vi "fgv_Gslam_history.vi"(7 "cmd":T1, 9 "z":dbl[][](array[numeric]), 10 "x_dr":cluster{"x":dbl, "y":dbl, "yaw":dbl}, 11 "x_true":cluster{"x":dbl, "y":dbl, "yaw":dbl}) -> (1 "hz":dbl[][][](array[numeric]), 2 "hxDR":cluster{"x":dbl, "y":dbl, "yaw":dbl}[](array[cluster]), 3 "hxTrue":cluster{"x":dbl, "y":dbl, "yaw":dbl}[](array[cluster]))   [LabVIEW 2019]
uses:
  Ctrl/mbuffer.ctl
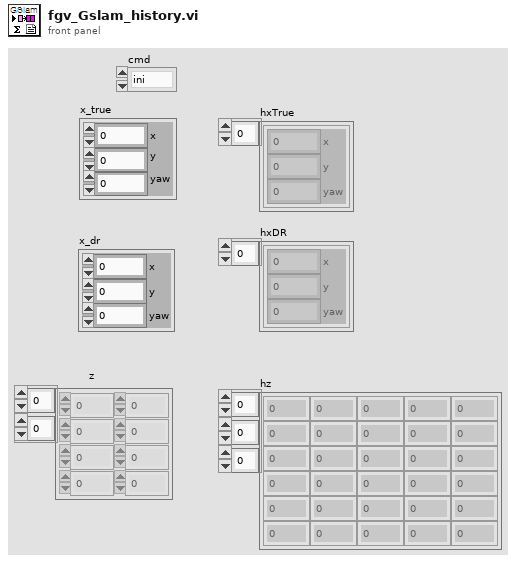
[diagram p1: front panel]
types:
  T1 = typedef "mbuffer.ctl" = enum16{"ini", "add", "read"}
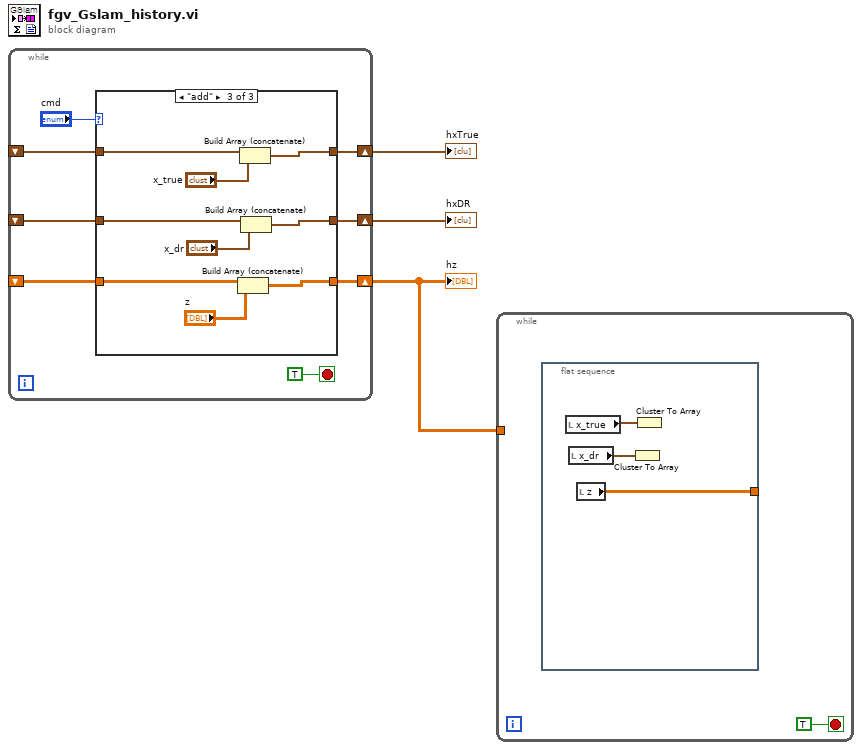
[diagram p0: block diagram]
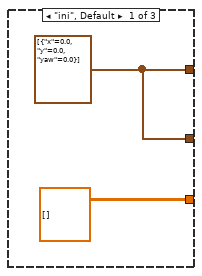
[diagram p2: hidden frame]
diagram:
  n1 = while {
    shift-right: [w10] -> w2
    shift-left: _ -> [w7]
    shift-right: [w9] -> w1
    shift-left: _ -> [w6]
    shift-right: [w8] -> w3
    shift-left: _ -> [w5]
    stop <- TRUE stop-if-true
    n2 = case shown="\"add\"" "cmd" {
      tunnel: [w13 w16 w23] -> w10
      tunnel: [w13 w15 w21] -> w9
      tunnel: [dbl[][][] [] w14 w18] -> w8
      tunnel: w7 -> [_ w16 w25]
      tunnel: w6 -> [_ w15 w22]
      tunnel: w5 -> [_ w14 w19]
      frame "ini", Default {
        w13 = cluster{"x":dbl, "y":dbl, "yaw":dbl}[] [{"x"=0.0, "y"=0.0, "yaw"=0.0}]
      }
      frame "read" {
      }
      frame "add" {
        n3 = Build Array (concatenate)(w19, "z") -> (w18:dbl[][][])
        n4 = Build Array (concatenate)(w25, "x_true") -> (w23:cluster{"x":dbl, "y":dbl, "yaw":dbl}[])
        n5 = Build Array (concatenate)(w22, "x_dr") -> (w21:cluster{"x":dbl, "y":dbl, "yaw":dbl}[])
      }
    }
  }
  "hz" <- w3
  "hxTrue" <- w2
  "hxDR" <- w1
  n6 = while {
    tunnel: w3 -> [_]
    stop <- TRUE stop-if-true
    n7 = flat-sequence {
      tunnel: [w27] -> _
      frame #0 {
        n8 = local read "x_true"() -> (w29:cluster{"x":dbl, "y":dbl, "yaw":dbl})
        n9 = local read "x_dr"() -> (w28:cluster{"x":dbl, "y":dbl, "yaw":dbl})
        n10 = local read "z"() -> (w27:dbl[][])
        n11 = Cluster To Array(cluster=w28) -> ()  [unwired: 1 out]
        n12 = Cluster To Array(cluster=w29) -> ()  [unwired: 1 out]
      }
    }
  }
